vi "Teleop.vi"(10 "Match Info":T1={"Autonomous Elapsed Seconds"=0.0, "TeleOp Elapsed Seconds"=0.0, "Disabled Elapsed Seconds"=0.0, "Visited Autonomous"=FALSE, "Visited TeleOp"=FALSE, "Visited Disabled"=FALSE, "Autonomous Settings"={"Autonomous Style"=enum."Independent", "VI Refnum"=refnum}}, 11 "Call Context":T2) -> ()   [LabVIEW 2016]
doc: "This VI is called for each TeleOp packet received from the DS where the robot is not disabled. It is often used to read from the joysticks and update I/O or to update setpoints for timed control loops. It should complete and return within 20 milliseconds or it may miss DS packets."
uses:
  <vilib>/Rock Robotics/WPI/DriverStation/WPI_DriverStationDerivedRobotMode.ctl
  <vilib>/Rock Robotics/WPI/DriverStation/WPI_DriverStationMatch Info.ctl
  <vilib>/Rock Robotics/WPI/ThirdParty/CanMotor/TalonSRX/WPI_CANTalonSRX_APIControlMode.ctl
  <vilib>/Rock Robotics/WPI/Relay/WPI_RelayValue.ctl
  <vilib>/Rock Robotics/WPI/Utilities/WPI_GetSetVariantRefNum.vi
  Robot Global Data.vi
  <vilib>/Rock Robotics/Network Tables/NT Read Number.vi
  <vilib>/Rock Robotics/Network Tables/NT Write Number.vi
  <vilib>/Rock Robotics/WPI/RobotDrive/WPI_RobotDriveMecanumDrive_Cartesian.vi
  <vilib>/Rock Robotics/Network Tables/NT Write Numeric Array.vi
panel:
  in  "LED Toggle":bool
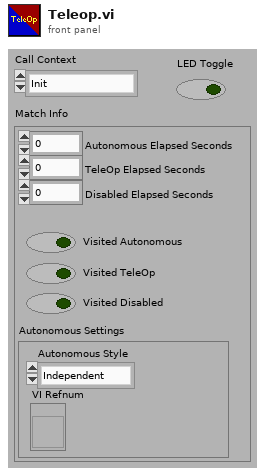
[diagram p1: front panel]
types:
  T1 = typedef "WPI_DriverStationMatch Info.ctl" = cluster{"Autonomous Elapsed Seconds":dbl, "TeleOp Elapsed Seconds":dbl, "Disabled Elapsed Seconds":dbl, "Visited Autonomous":bool, "Visited TeleOp":bool, "Visited Disabled":bool, "Autonomous Settings":cluster{"Autonomous Style":enum16{"Iterative", "Independent"}, "VI Refnum":refnum<vi>}}
  T2 = typedef "WPI_DriverStationDerivedRobotMode.ctl" = enum16{"Init", "Execute", "Stop"}
  T3 = typedef "WPI_CANTalonSRX_APIControlMode.ctl" = enum8{"Percent VBus", "Speed", "Position", "Slave", "Unchanged / Invalid", "Voltage Compensation", "Current", "Motion Profile", "Motion Magic"}
  T4 = typedef "WPI_JoystickDevRef.ctl" = cluster{"Device":T5}
  T5 = typedef "WPI_JoystickDeviceEnum.ctl" = enum16{"USB 0", "USB 1", "USB 2", "USB 3", "USB 4", "USB 5"}
  T6 = typedef "WPI_RelayDevRef.ctl" = cluster{"DevStatus":errorcluster, "Relay Channel":T7, "Relay Direction":T8}
  T7 = typedef "FPGA_DIORelayChannel.ctl" = enum8{"Relay 0", "Relay 1", "Relay 2", "Relay 3", "Invalid"}
  T8 = typedef "WPI_RelayDirection.ctl" = enum16{"Both directions", "Forward only", "Reverse only"}
  T9 = typedef "WPI_RelayValue.ctl" = enum16{"Off", "On", "Forward", "Reverse"}
  T10 = typedef "WPI_RobotDriveDevRef.ctl" = cluster{"DevStatus":errorcluster, "Motors[]":T11[], "Square Inputs":bool, "Max Output":dbl}
  T11 = typedef "WPI_MotorControlDeviceRef.ctl" = cluster{"DeviceStatus":errorcluster, "Type":T12, "PWM":cluster{"PWM Channel":T13, "DeadBand":T14}, "CAN":cluster{"Device Number":u8, "SetOutput VI Ref":variant, "GetOutput VI Ref":variant, "Enable VI Ref":variant, "Disable VI Ref":variant, "Data":variant}, "Invert":bool}
  T12 = typedef "WPI_MotorControlType.ctl" = enum16{"PWM", "CAN"}
  T13 = typedef "FPGA_DIOPWMChannel.ctl" = enum8{"PWM 0", "PWM 1", "PWM 2", "PWM 3", "PWM 4", "PWM 5", "PWM 6", "PWM 7", "PWM 8", "PWM 9", "PWM MXP 0", "PWM MXP 1", "PWM MXP 2", "PWM MXP 3", "PWM MXP 4", "PWM MXP 5", "PWM MXP 6", "PWM MXP 7", "PWM MXP 8", "PWM MXP 9", "Invalid"}
  T14 = typedef "WPI_PWMDeadband.ctl" = cluster{"Name":string, "maxPositivePwm":i32, "minPositivePwm":i32, "centerPwm":i32, "maxNegativePwm":i32, "minNegativePwm":i32, "angularRange":u16}
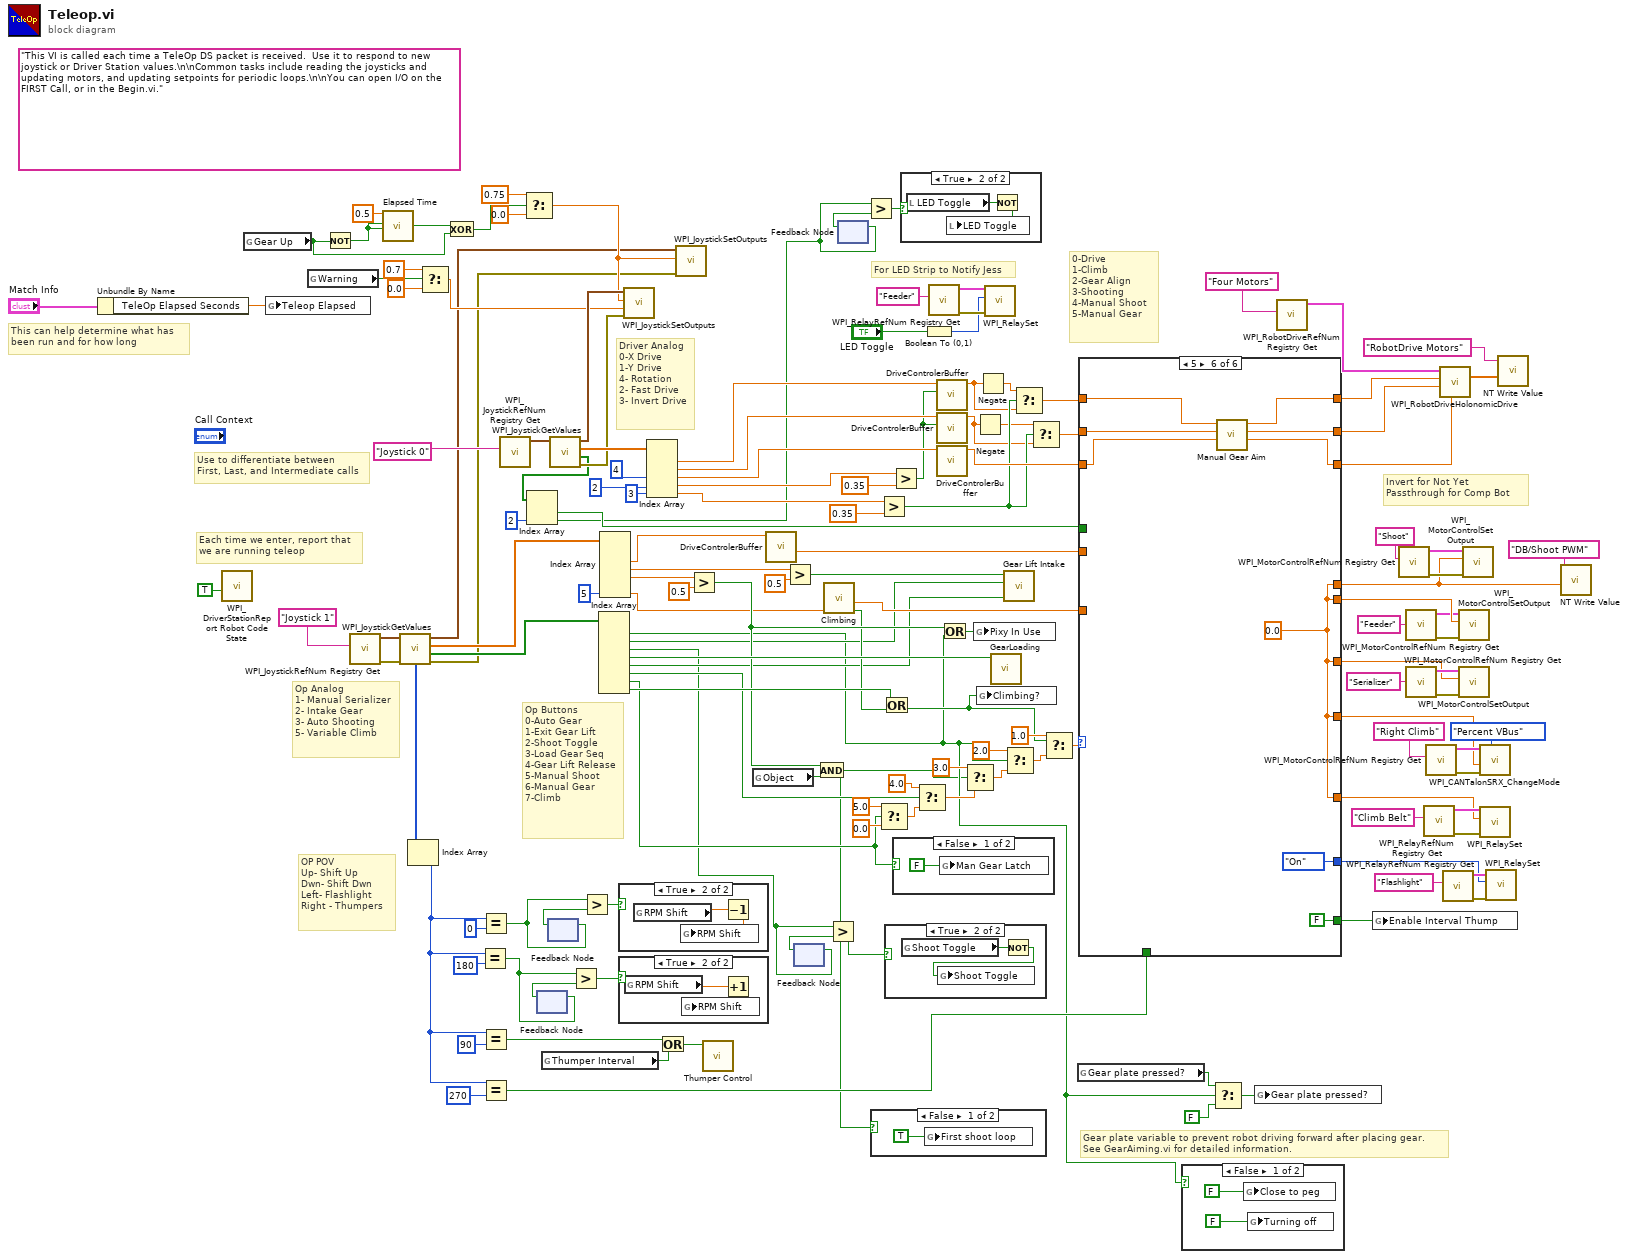
[diagram p0: block diagram]
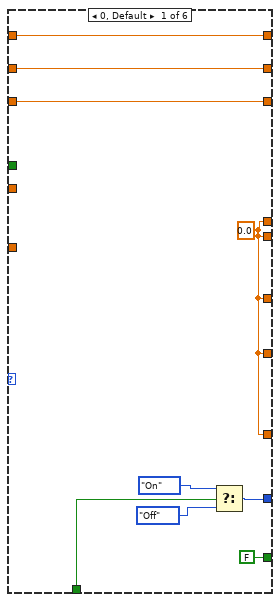
[diagram p9: hidden frame]
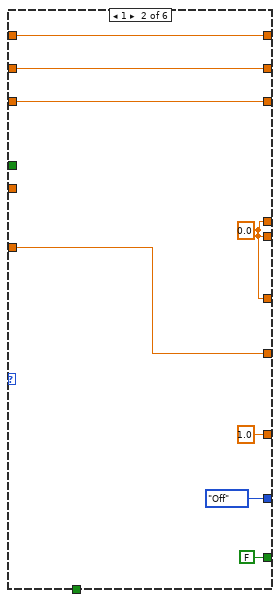
[diagram p10: hidden frame]
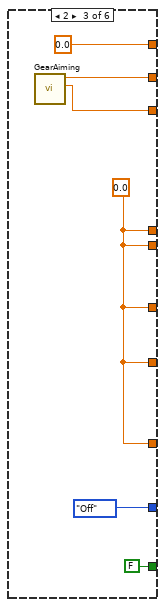
[diagram p11: hidden frame]
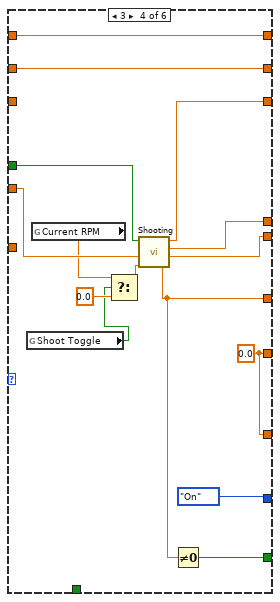
[diagram p12: hidden frame]
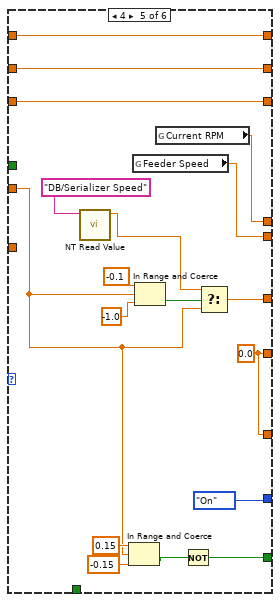
[diagram p13: hidden frame]
diagram:
  (unwired) "This VI is called each time a TeleOp DS packet is received.  Use it to respond to new joystick or Driver Station values.\n\nCommon tasks include reading the joysticks and updating motors, and updating setpoints for periodic loops.\n\nYou can open I/O on the FIRST Call, or in the Begin.vi."
  # "For LED Strip to Notify Jess"
  # "Gear plate variable to prevent robot driving forward after placing gear.\nSee GearAiming.vi for detailed information."
  # "OP POV \nUp- Shift Up\nDwn- Shift Dwn\nLeft- Flashlight\nRight - Thumpers"
  # "Invert for Not Yet\nPassthrough for Comp Bot"
  # "Op Analog\n1- Manual Serializer\n2- Intake Gear\n3- Auto Shooting\n5- Variable Climb"
  # "Op Buttons\n0-Auto Gear\n1-Exit Gear Lift\n2-Shoot Toggle\n3-Load Gear Seq\n4-Gear Lift Release\n5-Manual Shoot\n6-Manual Gear\n7-Climb"
  # "Driver Analog\n0-X Drive\n1-Y Drive\n4- Rotation\n2- Fast Drive\n3- Invert Drive"
  # "0-Drive\n1-Climb\n2-Gear Align\n3-Shooting\n4-Manual Shoot\n5-Manual Gear"
  # "Each time we enter, report that\nwe are running teleop"
  # "Use to differentiate between\nFirst, Last, and Intermediate calls"
  # "This can help determine what has\nbeen run and for how long"
  n1 = Unbundle By Name("Match Info") -> ("TeleOp Elapsed Seconds"=w70:dbl)
  n2 = call <vilib>:"WPI_DriverStationReport Robot Code State.vi"("TeleOp"=TRUE ("Autonomous")) -> ()  [unwired: 10 in, 1 out]
  n3 = global read "Robot Global Data.vi" "Gear Up"() -> (w21:bool)
  n4 = global write "Robot Global Data.vi" "Teleop Elapsed"(w70) -> ()
  n5 = global read "Robot Global Data.vi" "Warning"() -> (w55:bool)
  n6 = Not(x=w21) -> (.not. x?=w25:bool)
  n7 = call <vilib>:"WPI_JoystickRefNum Registry Get.vi"("refnum name"="Joystick 1") -> ("error out"=w27:errorcluster, "JoystickDevRef"=w124:T4)  [unwired: 1 in, 8 out]
  n8 = call "Elapsed Time"("Time Target (s)"=0.5, "Reset"=w25, "Auto Reset"=w25) -> ("Time has Elapsed"=w20:bool)  [unwired: 9 in, 7 out]
  n9 = call <vilib>:"WPI_JoystickGetValues.vi"("error in (no error)"=w27, "JoystickDevRef"=w124) -> ("error out"=w17:errorcluster, "Buttons"=w117:bool[], "Axes"=w105:dbl[], "JoystickDevRef"=w18:T4, "POVs"=w79:i16[])  [unwired: 5 in]
  n10 = Index Array(array=w79) -> (element=w40:i16)  [unwired: 1 in]
  n11 = Select(t=0.7, s=w55, f=0.0) -> (s? t:f=w45:dbl)
  n12 = Exclusive Or(1:w21, 2:w20) -> (0:w22:bool)
  n13 = Equal?(x=w40, y=i16 180) -> (x = y?=w71:bool)
  n14 = Equal?(x=w40, y=i16 0) -> (x = y?=w75:bool)
  n15 = Equal?(x=w40, y=i16 90) -> (x = y?=w33:bool)
  n16 = Equal?(x=w40, y=i16 270) -> (x = y?=w39:bool)
  n17 = call <vilib>:"WPI_JoystickRefNum Registry Get.vi"("refnum name"="Joystick 0") -> ("JoystickDevRef"=w143:T4)  [unwired: 1 in, 9 out]
  n18 = Select(t=0.75, s=w22, f=0.0) -> (s? t:f=w19:dbl)
  n19 = feedback #1() -> (w72:bool)  [unwired: 1 in]
  n20 = feedback-in #1(w71) -> ()
  n21 = global read "Robot Global Data.vi" "Thumper Interval"() -> (w32:bool)
  n22 = feedback-in #2(w75) -> ()
  n23 = feedback #2() -> (w74:bool)  [unwired: 1 in]
  n24 = call <vilib>:"WPI_JoystickGetValues.vi"("JoystickDevRef"=w143) -> ("error out"=w56:errorcluster, "Buttons"=w52:bool[], "Axes"=w141:dbl[], "JoystickDevRef"=w57:T4)  [unwired: 6 in, 1 out]
  n25 = Index Array(array=w52, index #2=2 ("index")) -> (element #1=w51:bool, element #2=w6:bool)  [unwired: 1 in]
  n26 = Greater?(x=w71, y=w72) -> (0:w73:bool)
  n27 = Greater?(x=w75, y=w74) -> (0:w76:bool)
  n28 = Index Array(array=w117) -> (element #1=w2:bool, element #2=w28:bool, element #3=w29:bool, element #4=w68:bool, element #5=w38:bool, element #6=w104:bool, element #7=w64:bool, element #8=w115:bool)  [unwired: 8 in]
  n29 = Index Array(array=w105, index #6=5 ("index")) -> (element #2=w101:dbl, element #3=w43:dbl, element #4=w103:dbl, element #6=w49:dbl)  [unwired: 5 in, 2 out]
  n30 = case shown="True" w76 {
    frame False {
    }
    frame True {
      n31 = global read "Robot Global Data.vi" "RPM Shift"() -> (w149:dbl)
      n32 = Decrement(x=w149) -> (x-1=w148:dbl)
      n33 = global write "Robot Global Data.vi" "RPM Shift"(w148) -> ()
    }
  }
  n34 = case shown="True" w73 {
    frame False {
    }
    frame True {
      n35 = global read "Robot Global Data.vi" "RPM Shift"() -> (w151:dbl)
      n36 = Increment(x=w151) -> (x+1=w150:dbl)
      n37 = global write "Robot Global Data.vi" "RPM Shift"(w150) -> ()
    }
  }
  n38 = call <vilib>:"WPI_JoystickSetOutputs.vi"("error in (no error)"=w56, "Right Rumble"=w45, "Left Rumble"=w19, "JoystickDevRef"=w57) -> ()  [unwired: 6 in, 2 out]
  n39 = Index Array(array=w141, index #3=4 ("index"), index #4=2 ("index"), index #5=3 ("index")) -> (element #1=w138:dbl, element #2=w137:dbl, element #3=w136:dbl, element #4=w122:dbl, element #5=w89:dbl)  [unwired: 2 in]
  n40 = Or(x=w33, y=w32) -> (x .or. y?=w35:bool)
  n41 = call <vilib>:"WPI_JoystickSetOutputs.vi"("error in (no error)"=w17, "Left Rumble"=w19, "JoystickDevRef"=w18) -> ()  [unwired: 7 in, 2 out]
  n42 = Greater?(x=w103, y=0.5) -> (0:w59:bool)
  n43 = call "Thumper Control.vi"("Thump"=w35) -> ()  [unwired: 11 in]
  n44 = global read "Robot Global Data.vi" "Object"() -> (w58:bool)
  n45 = call "DriveControlerBuffer.vi"("Input"=w101) -> ("Serializer Out"=w63:dbl)  [unwired: 9 in, 1 out]
  n46 = Greater?(x=w43, y=0.5) -> (0:w42:bool)
  n47 = feedback #3() -> (w31:bool)  [unwired: 1 in]
  n48 = feedback-in #3(w29) -> ()
  n49 = And(x=w59, y=w58) -> (x .and. y?=w1:bool)
  n50 = call "Climbing.vi"("Joystick In"=w49) -> ("Override"=w48:bool, "Climb Speed"=w47:dbl)  [unwired: 9 in]
  n51 = Greater?(x=w29, y=w31) -> (0:w30:bool)
  n52 = feedback #4() -> (w7:bool)  [unwired: 1 in]
  n53 = feedback-in #4(w6) -> ()
  n54 = Greater?(x=w6, y=w7) -> (0:w5:bool)
  n55 = case shown="False" w1 {
    frame False {
      n56 = global write "Robot Global Data.vi" "First shoot loop"(TRUE ("Latch")) -> ()
    }
    frame True {
    }
  }
  n57 = Greater?(x=w89, y=0.35) -> (0:w85:bool)
  n58 = Select(t=5.0, s=w64, f=0.0) -> (s? t:f=w66:dbl)
  n59 = Or(x=w115, y=w48) -> (x .or. y?=w16:bool)
  n60 = case shown="True" w30 {
    frame False {
    }
    frame True {
      n61 = global read "Robot Global Data.vi" "Shoot Toggle"() -> (w154:bool)
      n62 = Not(x=w154) -> (.not. x?=w153:bool)
      n63 = global write "Robot Global Data.vi" "Shoot Toggle"(w153) -> ()
    }
  }
  n64 = Greater?(x=w122, y=0.35) -> (0:w120:bool)
  n65 = case shown="False" w64 {
    frame False {
      n66 = global write "Robot Global Data.vi" "Man Gear Latch"(FALSE ("Latch")) -> ()
    }
    frame True {
    }
  }
  n67 = case shown="True" w5 {
    frame False {
    }
    frame True {
      n68 = local read "LED Toggle"() -> (w157:bool)
      n69 = Not(x=w157) -> (.not. x?=w156:bool)
      n70 = local write "LED Toggle"(w156) -> ()
    }
  }
  n71 = Select(t=4.0, s=w104, f=w66) -> (s? t:f=w119:dbl)
  n72 = Boolean To (0,1)(Boolean="LED Toggle") -> (0, 1=w4:i16)
  n73 = call <vilib>:"WPI_RelayRefNum Registry Get.vi"("refnum name"="Feeder") -> ("error out"=w10:errorcluster, "RelayDevRef"=w9:T6)  [unwired: 9 in]
  n74 = call "DriveControlerBuffer.vi"("Fast Drive"=w120, "Input"=w138) -> ("Drive Output"=w84:dbl)  [unwired: 8 in, 1 out]
  n75 = call "DriveControlerBuffer.vi"("Fast Drive"=w120, "Input"=w137) -> ("Drive Output"=w83:dbl)  [unwired: 8 in, 1 out]
  n76 = call "DriveControlerBuffer.vi"("Input"=w136) -> ("Drive Output"=w86:dbl)  [unwired: 9 in, 1 out]
  n77 = Or(x=w59, y=w2) -> (x .or. y?=w69:bool)
  n78 = Select(t=3.0, s=w1, f=w119) -> (s? t:f=w133:dbl)
  n79 = global write "Robot Global Data.vi" "Pixy In Use"(w69) -> ()
  n80 = Negate(x=w83) -> (-x=w81:dbl)
  n81 = global write "Robot Global Data.vi" "Climbing?"(w16) -> ()
  n82 = Negate(x=w84) -> (-x=w82:dbl)
  n83 = call <vilib>:"WPI_RelaySet.vi"("error in (no error)"=w10, "RelayValue"=w4, "RelayDevRef"=w9) -> ()  [unwired: 7 in, 2 out]
  n84 = call "GearLoading.vi"("Activate"=w68) -> ()  [unwired: 11 in]
  n85 = call "Gear Lift Intake.vi"("Release"=w38, "Exit Button"=w28, "Trigger"=w42) -> ()  [unwired: 9 in]
  n86 = Select(t=2.0, s=w2, f=w133) -> (s? t:f=w134:dbl)
  n87 = Select(t=w82, s=w85, f=w84) -> (s? t:f=w88:dbl)
  n88 = Select(t=w81, s=w85, f=w83) -> (s? t:f=w87:dbl)
  n89 = Select(t=1.0, s=w16, f=w134) -> (s? t:f=w135:dbl)
  n90 = global read "Robot Global Data.vi" "Gear plate pressed?"() -> (w60:bool)
  n91 = case shown="5" w135 {
    tunnel: [w166 w174 0.0 ("Output") w192 w213 w222] -> w129
    tunnel: w88 -> [w166 w174 _ w192 w213 w221]
    tunnel: [w165 w173 w179 w191 w212 w220] -> w126
    tunnel: w87 -> [w165 w173 _ w191 w212 w219]
    tunnel: [w164 w172 w178 w189 w211 w218] -> w128
    tunnel: w86 -> [w164 w172 _ _ w211 w217]
    tunnel: [w160 w171 w176 w195 w208 w216] -> w37
    tunnel: [w160 w171 w176 w188 w196 w216] -> w15
    tunnel: [w160 w168 w176 w193 w209 w216] -> w110
    tunnel: [w160 w171 w176 w182 w201 w216] -> w107
    tunnel: w63 -> [_ _ _ w190 w197 _]
    tunnel: [w162 WPI_RelayValue."Off" ("RelayValue") WPI_RelayValue."Off" ("RelayValue") WPI_RelayValue."On" ("RelayValue") WPI_RelayValue."On" ("RelayValue") WPI_RelayValue."On" ("RelayValue")] -> w98
    tunnel: [w160 1.0 ("Shooter Output") w176 w193 w209 w216] -> w93
    tunnel: w51 -> [_ _ _ w187 _ _]
    tunnel: w47 -> [_ w168 _ _ _ _]
    tunnel: w39 -> [w159 _ _ _ _ _]
    tunnel: [FALSE ("Thumper Out") FALSE ("Thumper Out") FALSE ("Thumper Out") w183 w198 FALSE ("Thumper Out")] -> w34
    frame 0, Default {
      w160 = 0.0 ("Shooter Output")
      n92 = Select(t=WPI_RelayValue."On", s=w159, f=WPI_RelayValue."Off" ("RelayValue")) -> (s? t:f=w162:T9)
    }
    frame 1 {
      w171 = 0.0 ("Shooter Output")
    }
    frame 2 {
      w176 = 0.0 ("Shooter Output")
      n93 = call "GearAiming.vi"() -> ("Drive Rotate"=w178:dbl, "Drive Y"=w179:dbl)  [unwired: 10 in]
    }
    frame 3 {
      w193 = 0.0 ("Shooter Output")
      n94 = global read "Robot Global Data.vi" "Shoot Toggle"() -> (w184:bool)
      n95 = global read "Robot Global Data.vi" "Current RPM"() -> (w181:dbl)
      n96 = Select(t=w181, s=w184, f=0.0) -> (s? t:f=w186:dbl)
      n97 = call "Shooting.vi"("Shoot override"=w186, "Serializer Override"=w190, "Lock PWM"=w187) -> ("Serializer Output"=w182:dbl, "Feeder Output"=w188:dbl, "Shooter \nPWM"=w195:dbl, "Rotation Out"=w189:dbl)  [unwired: 3 in]
      n98 = Not Equal To 0?(x=w182) -> (x != 0?=w183:bool)
    }
    frame 4 {
      w209 = 0.0 ("Shooter Output")
      n99 = call-poly <vilib>:"NT Read Value.vi"("Name"="DB/Serializer Speed") -> ("Numeric"=w204:dbl)  [unwired: 9 in, 1 out]
      n100 = In Range and Coerce(upper limit=0.15, x=w197, lower limit=-0.15) -> (In Range?=w202:bool)  [unwired: 1 out]
      n101 = global read "Robot Global Data.vi" "Feeder Speed"() -> (w196:dbl)
      n102 = In Range and Coerce(upper limit=-0.1, x=w197, lower limit=-1.0) -> (In Range?=w203:bool)  [unwired: 1 out]
      n103 = global read "Robot Global Data.vi" "Current RPM"() -> (w208:dbl)
      n104 = Not(x=w202) -> (.not. x?=w198:bool)
      n105 = Select(t=w204, s=w203, f=w197) -> (s? t:f=w201:dbl)
    }
    frame 5 {
      w216 = 0.0
      n106 = call "Manual Gear Aim.vi"("Rotate In"=w217, "Y In"=w219, "X Input"=w221) -> ("Rotate Out"=w218:dbl, "Y Out"=w220:dbl, "X Out"=w222:dbl)  [unwired: 6 in]
    }
  }
  n107 = case shown="False" w2 {
    frame False {
      n108 = global write "Robot Global Data.vi" "Close to peg"(FALSE ("Latch")) -> ()
      n109 = global write "Robot Global Data.vi" "Turning off"(FALSE ("Latch")) -> ()
    }
    frame True {
    }
  }
  n110 = Select(t=w60, s=w2, f=FALSE) -> (s? t:f=w62:bool)
  n111 = global write "Robot Global Data.vi" "Gear plate pressed?"(w62) -> ()
  n112 = call <vilib>:"WPI_RobotDriveRefNum Registry Get.vi"("refnum name"="Four Motors") -> ("RobotDriveDevRef"=w145:T10)  [unwired: 1 in, 9 out]
  n113 = global write "Robot Global Data.vi" "Enable Interval Thump"(w34) -> ()
  n114 = call <vilib>:"WPI_MotorControlRefNum Registry Get.vi"("refnum name"="Shoot") -> ("error out"=w80:errorcluster, "MotorControlDevRef"=w92:T11)  [unwired: 9 in]
  n115 = call <vilib>:"WPI_MotorControlRefNum Registry Get.vi"("refnum name"="Feeder") -> ("error out"=w12:errorcluster, "MotorControlDevRef"=w14:T11)  [unwired: 9 in]
  n116 = call <vilib>:"WPI_MotorControlRefNum Registry Get.vi"("refnum name"="Serializer") -> ("error out"=w109:errorcluster, "MotorControlDevRef"=w108:T11)  [unwired: 9 in]
  n117 = call <vilib>:"WPI_RelayRefNum Registry Get.vi"("refnum name"="Climb Belt") -> ("error out"=w96:errorcluster, "RelayDevRef"=w95:T6)  [unwired: 9 in]
  n118 = call <vilib>:"WPI_MotorControlRefNum Registry Get.vi"("refnum name"="Right Climb") -> ("error out"=w113:errorcluster, "MotorControlDevRef"=w112:T11)  [unwired: 9 in]
  n119 = call-poly <vilib>:"WPI_RobotDriveHolonomicDrive.vi"("Rotation"=w128, "Y"=w126, "X"=w129, "RobotDriveDevRef"=w145) -> ("Motor Values"=w139:dbl[])  [unwired: 5 in, 2 out]
  n120 = call <vilib>:"WPI_RelayRefNum Registry Get.vi"("refnum name"="Flashlight") -> ("error out"=w99:errorcluster, "RelayDevRef"=w100:T6)  [unwired: 9 in]
  n121 = call <vilib>:"WPI_MotorControlSetOutput.vi"("error in (no error)"=w12, "Output"=w15, "MotorControlDevRef"=w14) -> ()  [unwired: 6 in, 3 out]
  n122 = call <vilib>:"WPI_MotorControlSetOutput.vi"("error in (no error)"=w109, "Output"=w107, "MotorControlDevRef"=w108) -> ()  [unwired: 6 in, 3 out]
  n123 = call <vilib>:"WPI_MotorControlSetOutput.vi"("error in (no error)"=w80, "Output"=w37, "MotorControlDevRef"=w92) -> ()  [unwired: 6 in, 3 out]
  n124 = call <vilib>:"WPI_CANTalonSRX_ChangeMode.vi"("error in (no error)"=w113, "Output"=w110, "Control Mode"=WPI_CANTalonSRX_APIControlMode."Percent VBus", "CAN Talon SRX Ref"=w112) -> ()  [unwired: 6 in, 2 out]
  n125 = call <vilib>:"WPI_RelaySet.vi"("error in (no error)"=w96, "RelayValue"=w93, "RelayDevRef"=w95) -> ()  [unwired: 7 in, 2 out]
  n126 = call <vilib>:"WPI_RelaySet.vi"("error in (no error)"=w99, "RelayValue"=w98, "RelayDevRef"=w100) -> ()  [unwired: 7 in, 2 out]
  n127 = call-poly <vilib>:"NT Write Value.vi"("Numeric Array"=w139, "Name"="RobotDrive Motors") -> ()  [unwired: 9 in, 1 out]
  n128 = call-poly <vilib>:"NT Write Value.vi"("Numeric"=w37, "Name"="DB/Shoot PWM") -> ()  [unwired: 9 in, 1 out]
